vi "set_chart_width.vi"(10 "Values to Display":dbl=400.0, 11 "Ctl Refnum":refnum<vi>) -> ()   [LabVIEW 2016]
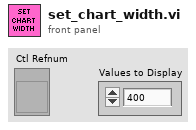
[diagram p1: front panel]
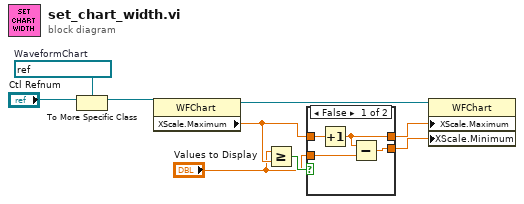
[diagram p0: block diagram]
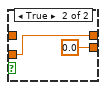
[diagram p2: hidden frame]
diagram:
  w2 = refnum<vi> refnum  # WaveformChart
  n1 = To More Specific Class(target class=w2, reference="Ctl Refnum") -> (specific class reference=w1:refnum<vi>)  [unwired: 1 in, 1 out]
  n2 = property on="Property Node" class="WFChart"(reference=w1) -> (reference out=w4:refnum<vi>, "XScale.Maximum"=w7:dbl)  [unwired: 1 in, 1 out]
  n3 = Greater Or Equal?(x="Values to Display", y=w7) -> (x >= y?=w6:bool)
  n4 = case shown="False" w6 {
    tunnel: "Values to Display" -> [w11 w15]
    tunnel: w7 -> [w13 _]
    tunnel: [w10 w15] -> w8
    tunnel: [w12 0.0] -> w9
    frame False {
      n5 = Increment(x=w13) -> (x+1=w10:dbl)
      n6 = Subtract(x=w10, y=w11) -> (x-y=w12:dbl)
    }
    frame True {
    }
  }
  n7 = property on="Property Node" class="WFChart"(reference=w4, "XScale.Maximum"=w8, "XScale.Minimum"=w9) -> ()  [unwired: 1 in, 2 out]
